vi "instance count allowed.vi"(8 "error in":errorcluster, 11 "Standard Engine Repo Data in":refnum<class "Standard Engine Configuration.lvclass">) -> (0 "error out":errorcluster, 2 "instances allowed (-1 = no limit)":i32, 3 "Standard Engine Repo Data out":refnum<class "Standard Engine Configuration.lvclass">)   [LabVIEW 2013, in "Standard Engine Configuration.lvclass"]
doc: "This property returns the number of instances of the execution code that can run on a target simultaneously."
uses:
  Standard Engine Configuration.lvclass
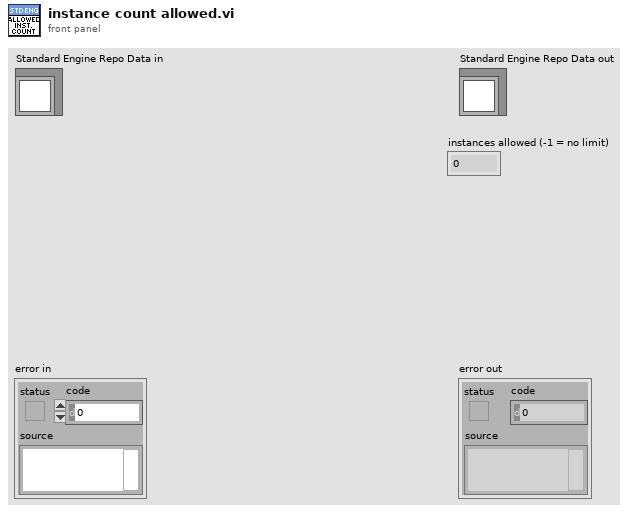
[diagram p1: front panel]
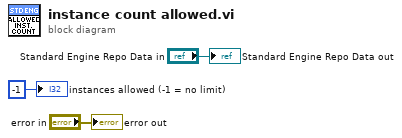
[diagram p0: block diagram]
diagram:
  "error out" <- "error in"
  "Standard Engine Repo Data out" <- "Standard Engine Repo Data in"
  "instances allowed (-1 = no limit)" <- -1 ("instances allowed (-1 = no limit)")
